vi "sync_auto_corr.vi"(8 "length":i32, 9 "delay":i32, 11 "samples in":cdb[](array[numeric])) -> (0 "autoVal":cdb[](array[numeric]), 3 "autoCorr":cdb[](array[numeric]))   [LabVIEW 2014]
panel:
  out "size(s)":i32
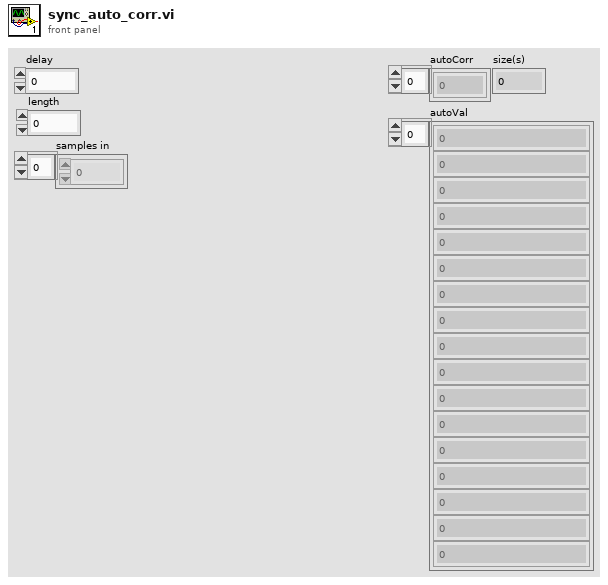
[diagram p1: front panel]
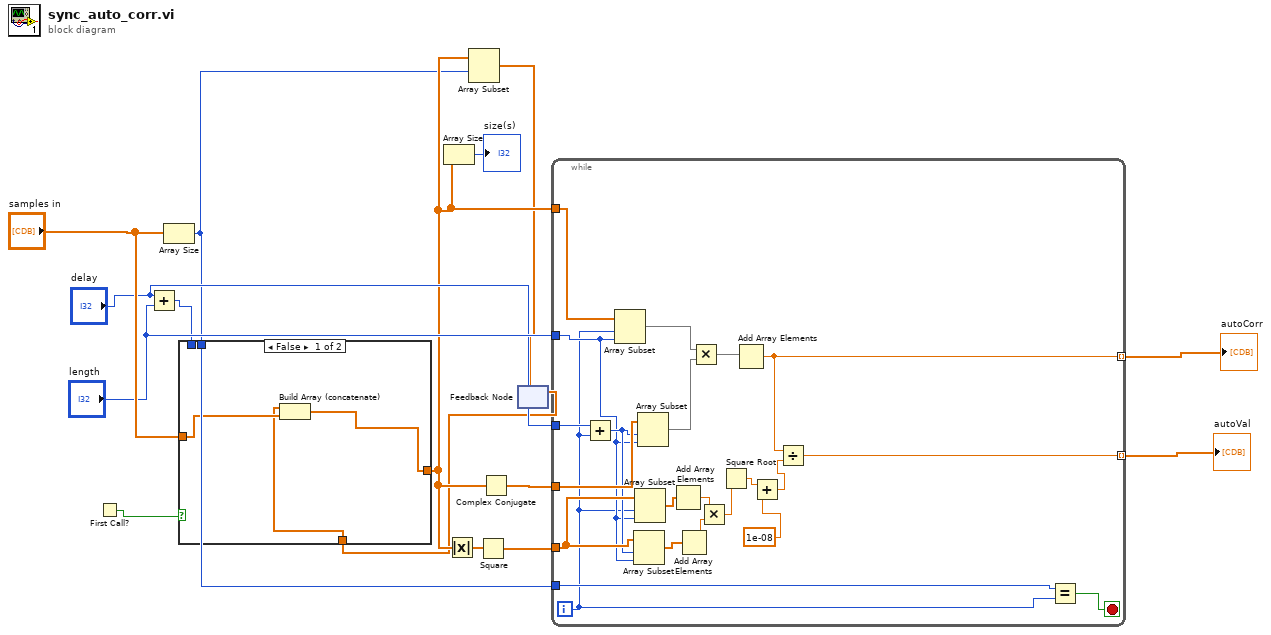
[diagram p0: block diagram]
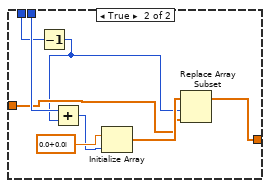
[diagram p2: hidden frame]
diagram:
  n1 = First Call?() -> (First Call?: T/F=w15:bool)
  n2 = Add(x="delay", y="length") -> (x+y=w4:i32)
  n3 = Array Size(array="samples in") -> (size(s)=w3:i32)
  n4 = feedback #1() -> (w1:cdb[])  [unwired: 1 in]
  n5 = case shown="False" w15 {
    tunnel: w3 -> [_ w26]
    tunnel: w4 -> [_ w20]
    tunnel: [w16 w21] -> w5
    tunnel: "samples in" -> [w18 w22]
    tunnel: w1 -> [w17 _]
    frame False {
      n6 = Build Array (concatenate)(w17, w18) -> (w16:cdb[])
    }
    frame True {
      n7 = Decrement(x=w20) -> (x-1=w19:i32)
      n8 = Add(x=w26, y=w19) -> (x+y=w24:i32)
      n9 = Initialize Array(cdb 0.0+0.0i, w24) -> (w23:cdb[])
      n10 = Replace Array Subset(array=w23, new element=w22, index=w19) -> (w21:cdb[])
    }
  }
  n11 = Array Size(array=w5) -> (size(s)=→"size(s)":i32)
  n12 = Absolute Value(x=w5) -> (abs(x)=w9:dbl[])
  n13 = Array Subset(array=w5, index=w3) -> (w2:cdb[])  [unwired: 1 in]
  n14 = Square(x=w9) -> (x^2=w8:dbl[])
  n15 = Complex Conjugate(1:w5) -> (0:w12:cdb[])
  n16 = feedback-in #1(w2) -> ()
  n17 = while {
    tunnel: w3 -> [w48]
    tunnel: "length" -> [w39]
    tunnel: w12 -> [w46]
    tunnel: "delay" -> [w45]
    tunnel: [w38] -> w10 mode=indexing
    tunnel: w8 -> [w41]
    tunnel: [w37] -> w7 mode=indexing
    tunnel: w5 -> [w27]
    i -> [w28]
    stop <- w47 stop-if-true
    n18 = Add(x=w45, y=w28) -> (x+y=w40:i32)
    n19 = Array Subset(array=w27, index=w28, length=w39) -> (w44:cdb[])
    n20 = Array Subset(array=w41, index=w40, length=w39) -> (w35:dbl[])
    n21 = Array Subset(array=w41, index=w28, length=w39) -> (w36:dbl[])
    n22 = Array Subset(array=w46, index=w40, length=w39) -> (w43:cdb[])
    n23 = Add Array Elements(numeric array=w36) -> (sum=w34:dbl)
    n24 = Add Array Elements(numeric array=w35) -> (sum=w33:dbl)
    n25 = Multiply(x=w44, y=w43) -> (x*y=w42:cdb[])
    n26 = Multiply(x=w34, y=w33) -> (x*y=w32:dbl)
    n27 = Square Root(x=w32) -> (sqrt(x)=w31:dbl)
    n28 = Add Array Elements(numeric array=w42) -> (sum=w38:cdb)
    n29 = Add(x=w31, y=1e-08) -> (x+y=w29:dbl)
    n30 = Divide(x=w38, y=w29) -> (x/y=w37:cdb)
    n31 = Equal?(x=w48, y=w28) -> (x = y?=w47:bool)
  }
  "autoCorr" <- w10
  "autoVal" <- w7
